vi "FPGANic.Globals.vi"() -> ()   [LabVIEW 2017]
panel:
  out "FPGA VI Reference Out":refnum<k20>
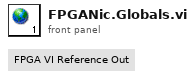
[diagram p1: front panel]
diagram:
